vi "Wait for spectrometer_v2.vi"(8 "error in (no error)":errorcluster, 11 "VISA Refnum in":refnum<visa-resource-name>) -> (0 "error out":errorcluster, 2 "SRQ 1 Control Value":u16, 3 "VISA Refnum out":refnum<visa-resource-name>)   [LabVIEW 2018]
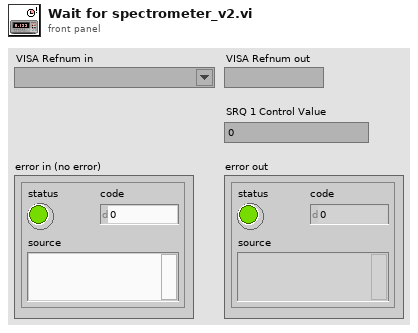
[diagram p1: front panel]
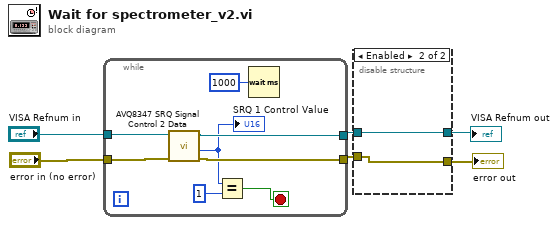
[diagram p0: block diagram]
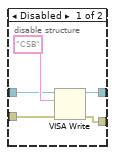
[diagram p2: hidden frame]
diagram:
  n1 = while {
    tunnel: "VISA Refnum in" -> [w12]
    tunnel: "error in (no error)" -> [w11]
    tunnel: [w9] -> w4
    tunnel: [w10] -> w3
    stop <- w13 stop-if-true
    n2 = call "AVQ8347 SRQ Signal Control 2 Data.vi"("Error In"=w11, "VISA Session"=w12) -> ("Error Out"=w10:errorcluster, "SRQ 2 Control Value"=w8:u16, "Copy VISA Session"=w9:refnum<visa-resource-name>)  [unwired: 6 in, 1 out]
    "SRQ 1 Control Value" <- w8
    n3 = Equal?(x=w8, y=u16 1) -> (x = y?=w13:bool)
    n4 = Wait (ms)(milliseconds to wait=u32 1000) -> ()  [unwired: 1 out]
  }
  n5 = disable-structure shown="Enabled" {
    disable-tunnel: w4 -> [w18 w21]
    disable-tunnel: w3 -> [w17 w20]
    disable-tunnel: [w16 w21] -> w2
    disable-tunnel: [w15 w20] -> w1
    frame Disabled {
      n6 = VISA Write(VISA resource name=w18, write buffer="CSB", error in (no error)=w17) -> (VISA resource name out=w16:refnum<visa-resource-name>, error out=w15:errorcluster)  [unwired: 1 out]
    }
    frame Enabled {
    }
  }
  "error out" <- w1
  "VISA Refnum out" <- w2
